vi "Self Test.vi"(8 "error in":errorcluster, 11 "34980A in":refnum<class "34980A.lvclass">) -> (0 "error out":errorcluster, 3 "34980A out":refnum<class "34980A.lvclass">)   [LabVIEW 2019, in "34980A.lvlib" / "34980A.lvclass"]
doc: "This Override VI must be called by ancestor classes\nThis class reads error data and transmits it to the fault handler"
uses:
  Library/34980A.lvclass
  Library/34980A.lvclass/34980A.ctl
  builds/Instruments/MLTFNC.lvlibp/Library/MLTFNC.lvclass
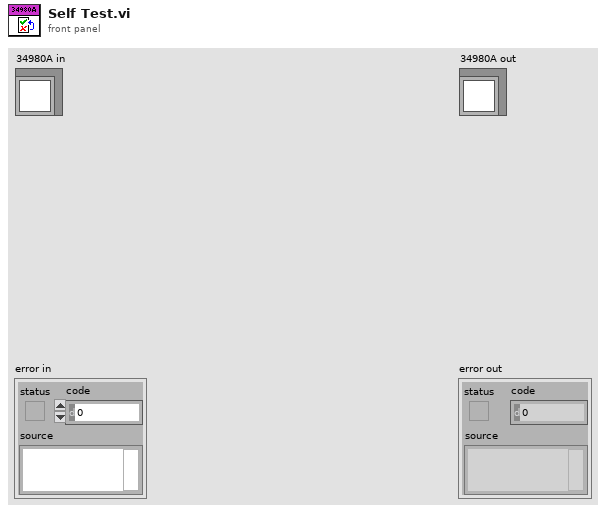
[diagram p1: front panel]
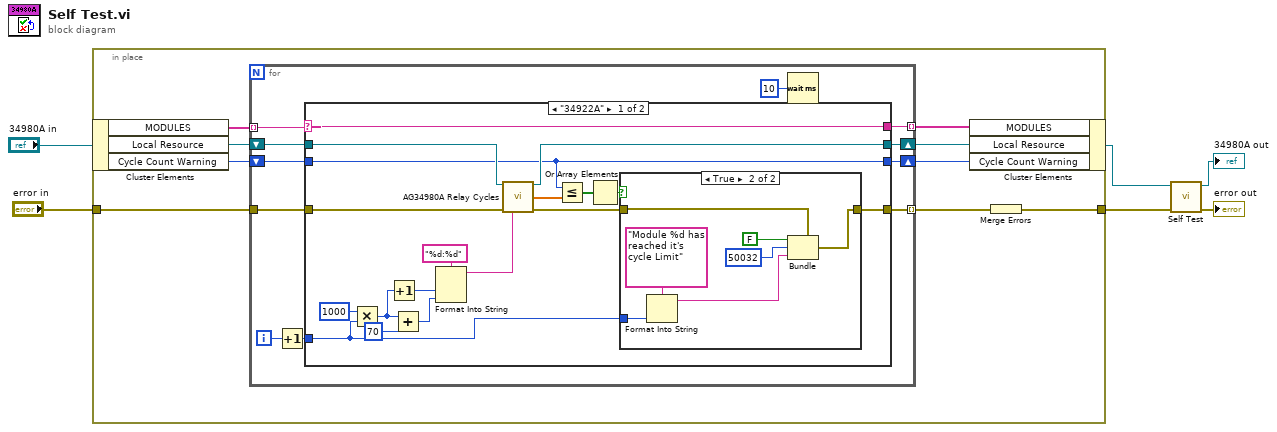
[diagram p0: block diagram]
diagram:
  n1 = in-place {
    in-place-border: "error in" -> [w11]
    in-place-border: [w7] -> w1
    n2 = in-place-cluster #1("34980A in") -> ("MODULES"=w15:string[], "Local Resource"=w13:refnum<visa-resource-name>, "Cycle Count Warning"=w12:u32)
    n3 = for {
      tunnel: w15 -> [w26] mode=indexing
      tunnel: [w25] -> w14 mode=indexing
      shift-right: [w22] -> w8
      shift-left: w13 -> [w24]
      shift-right: [w21] -> w9
      shift-left: w12 -> [w23]
      tunnel: w11 -> [w20]
      tunnel: [w19] -> w10 mode=indexing
      i -> [w18]
      n4 = Increment(x=w18) -> (x+1=w17:i32)
      n5 = case shown="\"34922A\"" w26 {
        selector: w26 -> [w44 w56]
        tunnel: [w44 w56] -> w25
        tunnel: w24 -> [w43 w55]
        tunnel: w23 -> [w39 w54]
        tunnel: [w42 w55] -> w22
        tunnel: [w39 w54] -> w21
        tunnel: w20 -> [w41 w53]
        tunnel: [w35 w53] -> w19
        tunnel: w17 -> [w34 _]
        frame "34922A" {
          n6 = Multiply(x=1000, y=w34) -> (x*y=w31:i32)
          n7 = Increment(x=w31) -> (x+1=w30:i32)
          n8 = Add(x=w31, y=70) -> (x+y=w29:i32)
          n9 = Format Into String(format string="%d:%d", w30, w29) -> (resulting string=w27:string)  [unwired: 2 in, 1 out]
          n10 = call <instrlib>:"AG34980A Relay Cycles.vi"("VISA resource name"=w43, "Channel List(empty)"=w27, "error in (no error)"=w41) -> ("VISA resource name out"=w42:refnum<visa-resource-name>, "Cycles"=w40:dbl[], "error out"=w36:errorcluster)  [unwired: 10 in]
          n11 = Less Or Equal?(x=w39, y=w40) -> (x <= y?=w38:bool[])
          n12 = Or Array Elements(Boolean array=w38) -> (logical OR=w37:bool)
          n13 = case shown="True" w37 {
            tunnel: w36 -> [w45 w52]
            tunnel: [w45 w46] -> w35
            tunnel: w34 -> [_ w48]
            frame False {
            }
            frame True {
              n14 = Format Into String(format string="Module %d has reached it's cycle Limit", w48) -> (resulting string=w47:string)  [unwired: 2 in, 1 out]
              n15 = Bundle(cluster=w52, "status"=FALSE, "code"=50032, "source"=w47) -> (w46:errorcluster)
            }
          }
        }
        frame Default {
        }
      }
      n16 = Wait (ms)(milliseconds to wait=u32 10) -> ()  [unwired: 1 out]
    }
    n17 = in-place-cluster #1("MODULES"=w14, "Local Resource"=w8, "Cycle Count Warning"=w9) -> (w2:refnum<class "34980A.lvclass">)
    n18 = Merge Errors(w10) -> (w7:errorcluster)
  }
  n19 = call-parent "Self Test.vi"("error in"=w1, "Instruments in"=w2) -> ("error out"=→"error out":errorcluster, "Instruments out"=→"34980A out":refnum<class "34980A.lvclass">)  [unwired: 8 in]
